vi "Calculator-test_harness.vi"(11 "test case ID":string) -> (3 "result":bool)   [LabVIEW 2015]
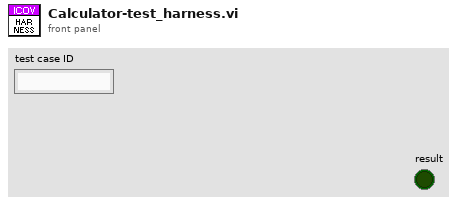
[diagram p1: front panel]
types:
  T1 = typedef "Operation.ctl" = enum16{"Add", "Subtract", "Multiply", "Divide"}
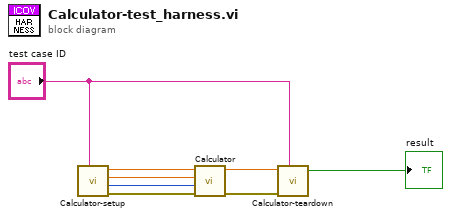
[diagram p0: block diagram]
diagram:
  n1 = call "Calculator-setup.vi"("test case ID"="test case ID") -> ("error in (no error)"=w3:errorcluster, "Operation"=w4:T1, "b"=w5:dbl, "a"=w6:dbl)  [unwired: 7 in]
  n2 = call "Calculator.vi"("error in (no error)"=w3, "Operation"=w4, "b"=w5, "a"=w6) -> ("error out"=w1:errorcluster, "result"=w2:dbl)  [unwired: 6 in]
  n3 = call "Calculator-teardown.vi"("test case ID"="test case ID", "error in (no error)"=w1, "result"=w2) -> ("result"=→"result":bool)  [unwired: 8 in]
